vi "communication manager.vi"() -> ()   [LabVIEW 2018]
uses:
  communication-manager/socket REP/socket REP.lvclass
  C:/Users/Denis/Desktop/S4CCS/S4CCS/communication-manager/Socket/Socket.lvclass
  communication-manager/socket SUB/socket SUB.lvclass
  communication-manager/socket PUB/socket PUB.lvclass
  communication-manager/RxTx/RxTx.lvclass
  <vilib>/addons/zeromq/zmq_context.lvclass
  communication-manager/Socket/Socket.lvclass
panel:
  out "error out":errorcluster
  in  "socket PUB.lvclass":refnum<class "socket PUB.lvclass">
  in  "socket SUB.lvclass":refnum<class "socket SUB.lvclass">
  in  "socket REP.lvclass":refnum<class "socket REP.lvclass">
  # "Communication Manager of S4CCS"
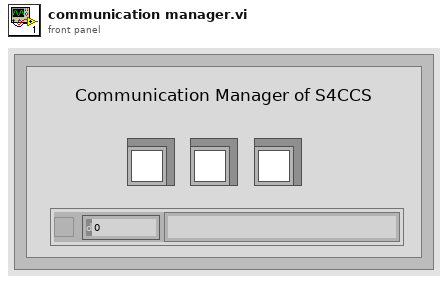
[diagram p1: front panel]
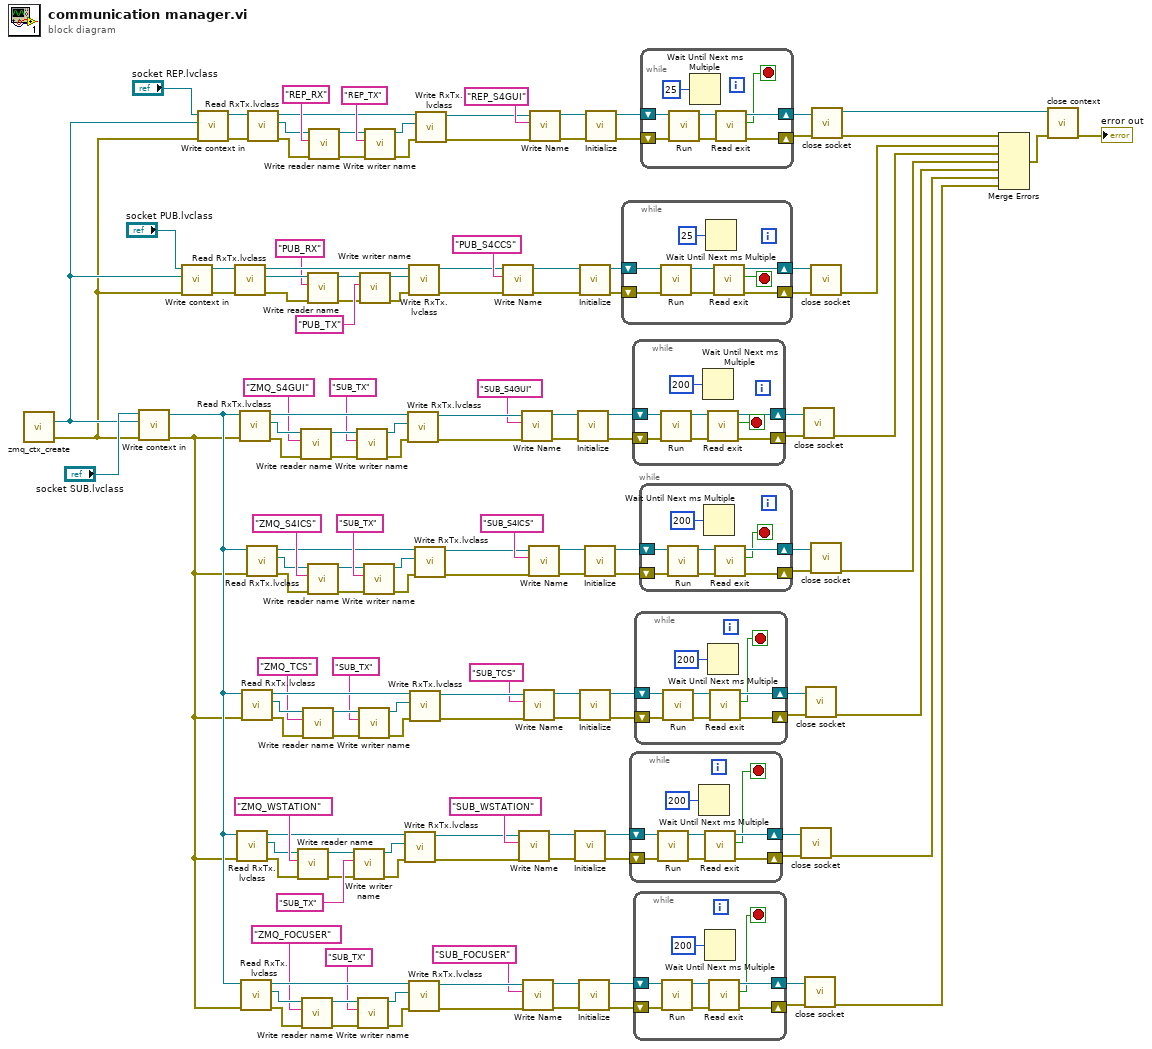
[diagram p0: block diagram]
diagram:
  n1 = call <vilib>:"zmq_ctx_create.vi"() -> ("error out"=w3:errorcluster, "context out"=w4:refnum<class "zmq_context.lvclass">)  [unwired: 4 in]
  n2 = call-dynamic "Write context in.vi"("error in (no error)"=w3, "zeromq.lvlib:ZeroMQ Context"=w4, "Socket in"="socket SUB.lvclass") -> ("error out"=w1:errorcluster, "Socket out"=w2:refnum<class "socket SUB.lvclass">)  [unwired: 7 in]
  n3 = call-dynamic "Write context in.vi"("error in (no error)"=w3, "zeromq.lvlib:ZeroMQ Context"=w4, "Socket in"="socket PUB.lvclass") -> ("error out"=w7:errorcluster, "Socket out"=w8:refnum<class "socket PUB.lvclass">)  [unwired: 7 in]
  n4 = call-dynamic "Write context in.vi"("error in (no error)"=w3, "zeromq.lvlib:ZeroMQ Context"=w4, "Socket in"="socket REP.lvclass") -> ("error out"=w10:errorcluster, "Socket out"=w11:refnum<class "socket REP.lvclass">)  [unwired: 7 in]
  n5 = call-dynamic "Read RxTx.lvclass.vi"("error in (no error)"=w7, "Socket in"=w8) -> ("error out"=w116:errorcluster, "RxTx.lvclass"=w120:refnum<class "RxTx.lvclass">, "Socket out"=w117:refnum<class "socket PUB.lvclass">)  [unwired: 7 in]
  n6 = call-dynamic "Read RxTx.lvclass.vi"("error in (no error)"=w1, "Socket in"=w2) -> ("error out"=w51:errorcluster, "RxTx.lvclass"=w55:refnum<class "RxTx.lvclass">, "Socket out"=w52:refnum<class "socket SUB.lvclass">)  [unwired: 7 in]
  n7 = call-dynamic "Read RxTx.lvclass.vi"("error in (no error)"=w1, "Socket in"=w2) -> ("error out"=w98:errorcluster, "RxTx.lvclass"=w94:refnum<class "RxTx.lvclass">, "Socket out"=w97:refnum<class "socket SUB.lvclass">)  [unwired: 7 in]
  n8 = call-dynamic "Read RxTx.lvclass.vi"("error in (no error)"=w1, "Socket in"=w2) -> ("error out"=w32:errorcluster, "RxTx.lvclass"=w28:refnum<class "RxTx.lvclass">, "Socket out"=w31:refnum<class "socket SUB.lvclass">)  [unwired: 7 in]
  n9 = call-dynamic "Read RxTx.lvclass.vi"("error in (no error)"=w1, "Socket in"=w2) -> ("error out"=w64:errorcluster, "RxTx.lvclass"=w60:refnum<class "RxTx.lvclass">, "Socket out"=w63:refnum<class "socket SUB.lvclass">)  [unwired: 7 in]
  n10 = call-dynamic "Read RxTx.lvclass.vi"("error in (no error)"=w1, "Socket in"=w2) -> ("error out"=w83:errorcluster, "RxTx.lvclass"=w87:refnum<class "RxTx.lvclass">, "Socket out"=w84:refnum<class "socket SUB.lvclass">)  [unwired: 7 in]
  n11 = call-dynamic "Read RxTx.lvclass.vi"("error in (no error)"=w10, "Socket in"=w11) -> ("error out"=w140:errorcluster, "RxTx.lvclass"=w144:refnum<class "RxTx.lvclass">, "Socket out"=w141:refnum<class "socket REP.lvclass">)  [unwired: 7 in]
  n12 = call-dynamic "Write reader name.vi"("error in (no error)"=w51, "RX name"="ZMQ_WSTATION" ("reader name"), "RxTx in"=w55) -> ("error out"=w50:errorcluster, "RxTx out"=w54:refnum<class "RxTx.lvclass">)  [unwired: 7 in]
  n13 = call-dynamic "Write reader name.vi"("error in (no error)"=w98, "RX name"="ZMQ_S4GUI" ("reader name"), "RxTx in"=w94) -> ("error out"=w99:errorcluster, "RxTx out"=w95:refnum<class "RxTx.lvclass">)  [unwired: 7 in]
  n14 = call-dynamic "Write reader name.vi"("error in (no error)"=w32, "RX name"="ZMQ_FOCUSER" ("reader name"), "RxTx in"=w28) -> ("error out"=w33:errorcluster, "RxTx out"=w29:refnum<class "RxTx.lvclass">)  [unwired: 7 in]
  n15 = call-dynamic "Write reader name.vi"("error in (no error)"=w64, "RX name"="ZMQ_TCS" ("reader name"), "RxTx in"=w60) -> ("error out"=w65:errorcluster, "RxTx out"=w61:refnum<class "RxTx.lvclass">)  [unwired: 7 in]
  n16 = call-dynamic "Write reader name.vi"("error in (no error)"=w116, "RX name"="PUB_RX" ("reader name"), "RxTx in"=w120) -> ("error out"=w115:errorcluster, "RxTx out"=w119:refnum<class "RxTx.lvclass">)  [unwired: 7 in]
  n17 = call-dynamic "Write reader name.vi"("error in (no error)"=w83, "RX name"="ZMQ_S4ICS" ("reader name"), "RxTx in"=w87) -> ("error out"=w82:errorcluster, "RxTx out"=w86:refnum<class "RxTx.lvclass">)  [unwired: 7 in]
  n18 = call-dynamic "Write reader name.vi"("error in (no error)"=w140, "RX name"="REP_RX" ("reader name"), "RxTx in"=w144) -> ("error out"=w139:errorcluster, "RxTx out"=w143:refnum<class "RxTx.lvclass">)  [unwired: 7 in]
  n19 = call-dynamic "Write writer name.vi"("error in (no error)"=w50, "Tx name"="SUB_TX" ("writer name"), "RxTx in"=w54) -> ("error out"=w49:errorcluster, "RxTx out"=w53:refnum<class "RxTx.lvclass">)  [unwired: 7 in]
  n20 = call-dynamic "Write writer name.vi"("error in (no error)"=w99, "Tx name"="SUB_TX" ("writer name"), "RxTx in"=w95) -> ("error out"=w100:errorcluster, "RxTx out"=w96:refnum<class "RxTx.lvclass">)  [unwired: 7 in]
  n21 = call-dynamic "Write writer name.vi"("error in (no error)"=w33, "Tx name"="SUB_TX" ("writer name"), "RxTx in"=w29) -> ("error out"=w34:errorcluster, "RxTx out"=w30:refnum<class "RxTx.lvclass">)  [unwired: 7 in]
  n22 = call-dynamic "Write writer name.vi"("error in (no error)"=w65, "Tx name"="SUB_TX" ("writer name"), "RxTx in"=w61) -> ("error out"=w66:errorcluster, "RxTx out"=w62:refnum<class "RxTx.lvclass">)  [unwired: 7 in]
  n23 = call-dynamic "Write writer name.vi"("error in (no error)"=w115, "Tx name"="PUB_TX" ("writer name"), "RxTx in"=w119) -> ("error out"=w114:errorcluster, "RxTx out"=w118:refnum<class "RxTx.lvclass">)  [unwired: 7 in]
  n24 = call-dynamic "Write writer name.vi"("error in (no error)"=w82, "Tx name"="SUB_TX" ("writer name"), "RxTx in"=w86) -> ("error out"=w81:errorcluster, "RxTx out"=w85:refnum<class "RxTx.lvclass">)  [unwired: 7 in]
  n25 = call-dynamic "Write writer name.vi"("error in (no error)"=w139, "Tx name"="REP_TX" ("writer name"), "RxTx in"=w143) -> ("error out"=w138:errorcluster, "RxTx out"=w142:refnum<class "RxTx.lvclass">)  [unwired: 7 in]
  n26 = call-dynamic "Write RxTx.lvclass.vi"("error in (no error)"=w49, "RxTx.lvclass"=w53, "Socket in"=w52) -> ("error out"=w46:errorcluster, "Socket out"=w47:refnum<class "socket SUB.lvclass">)  [unwired: 7 in]
  n27 = call-dynamic "Write RxTx.lvclass.vi"("error in (no error)"=w100, "RxTx.lvclass"=w96, "Socket in"=w97) -> ("error out"=w103:errorcluster, "Socket out"=w102:refnum<class "socket SUB.lvclass">)  [unwired: 7 in]
  n28 = call-dynamic "Write RxTx.lvclass.vi"("error in (no error)"=w114, "RxTx.lvclass"=w118, "Socket in"=w117) -> ("error out"=w12:errorcluster, "Socket out"=w13:refnum<class "socket PUB.lvclass">)  [unwired: 7 in]
  n29 = call-dynamic "Write RxTx.lvclass.vi"("error in (no error)"=w34, "RxTx.lvclass"=w30, "Socket in"=w31) -> ("error out"=w37:errorcluster, "Socket out"=w36:refnum<class "socket SUB.lvclass">)  [unwired: 7 in]
  n30 = call-dynamic "Write RxTx.lvclass.vi"("error in (no error)"=w66, "RxTx.lvclass"=w62, "Socket in"=w63) -> ("error out"=w69:errorcluster, "Socket out"=w68:refnum<class "socket SUB.lvclass">)  [unwired: 7 in]
  n31 = call-dynamic "Write RxTx.lvclass.vi"("error in (no error)"=w81, "RxTx.lvclass"=w85, "Socket in"=w84) -> ("error out"=w78:errorcluster, "Socket out"=w79:refnum<class "socket SUB.lvclass">)  [unwired: 7 in]
  n32 = call-dynamic "Write RxTx.lvclass.vi"("error in (no error)"=w138, "RxTx.lvclass"=w142, "Socket in"=w141) -> ("error out"=w135:errorcluster, "Socket out"=w136:refnum<class "socket REP.lvclass">)  [unwired: 7 in]
  n33 = call-dynamic "Write Name.vi"("error in (no error)"=w12, "Name"="PUB_S4CCS", "Socket in"=w13) -> ("error out"=w112:errorcluster, "Socket out"=w113:refnum<class "socket PUB.lvclass">)  [unwired: 7 in]
  n34 = call-dynamic "Write Name.vi"("error in (no error)"=w46, "Name"="SUB_WSTATION", "Socket in"=w47) -> ("error out"=w20:errorcluster, "Socket out"=w21:refnum<class "socket SUB.lvclass">)  [unwired: 7 in]
  n35 = call-dynamic "Write Name.vi"("error in (no error)"=w103, "Name"="SUB_S4GUI", "Socket in"=w102) -> ("error out"=w18:errorcluster, "Socket out"=w19:refnum<class "socket SUB.lvclass">)  [unwired: 7 in]
  n36 = call-dynamic "Write Name.vi"("error in (no error)"=w37, "Name"="SUB_FOCUSER", "Socket in"=w36) -> ("error out"=w14:errorcluster, "Socket out"=w15:refnum<class "socket SUB.lvclass">)  [unwired: 7 in]
  n37 = call-dynamic "Write Name.vi"("error in (no error)"=w69, "Name"="SUB_TCS", "Socket in"=w68) -> ("error out"=w24:errorcluster, "Socket out"=w25:refnum<class "socket SUB.lvclass">)  [unwired: 7 in]
  n38 = call-dynamic "Write Name.vi"("error in (no error)"=w78, "Name"="SUB_S4ICS", "Socket in"=w79) -> ("error out"=w22:errorcluster, "Socket out"=w23:refnum<class "socket SUB.lvclass">)  [unwired: 7 in]
  n39 = call-dynamic "Write Name.vi"("error in (no error)"=w135, "Name"="REP_S4GUI", "Socket in"=w136) -> ("error out"=w16:errorcluster, "Socket out"=w17:refnum<class "socket REP.lvclass">)  [unwired: 7 in]
  n40 = call-dynamic "Initialize.vi"("error in (no error)"=w20, "socket SUB in"=w21) -> ("error out"=w43:errorcluster, "socket SUB out"=w45:refnum<class "socket SUB.lvclass">)  [unwired: 8 in]
  n41 = call-dynamic "Initialize.vi"("error in (no error)"=w18, "socket SUB in"=w19) -> ("error out"=w106:errorcluster, "socket SUB out"=w104:refnum<class "socket SUB.lvclass">)  [unwired: 8 in]
  n42 = call-dynamic "Initialize.vi"("error in (no error)"=w14, "socket SUB in"=w15) -> ("error out"=w40:errorcluster, "socket SUB out"=w38:refnum<class "socket SUB.lvclass">)  [unwired: 8 in]
  n43 = call-dynamic "Initialize.vi"("error in (no error)"=w112, "socket PUB in"=w113) -> ("error out"=w109:errorcluster, "socket PUB out"=w111:refnum<class "socket PUB.lvclass">)  [unwired: 8 in]
  n44 = call-dynamic "Initialize.vi"("error in (no error)"=w24, "socket SUB in"=w25) -> ("error out"=w72:errorcluster, "socket SUB out"=w70:refnum<class "socket SUB.lvclass">)  [unwired: 8 in]
  n45 = call-dynamic "Initialize.vi"("error in (no error)"=w22, "socket SUB in"=w23) -> ("error out"=w75:errorcluster, "socket SUB out"=w77:refnum<class "socket SUB.lvclass">)  [unwired: 8 in]
  n46 = call-dynamic "Initialize.vi"("error in (no error)"=w16, "socket REP in"=w17) -> ("error out"=w132:errorcluster, "socket REP out"=w134:refnum<class "socket REP.lvclass">)  [unwired: 8 in]
  n47 = while {
    shift-right: [w151] -> w110
    shift-left: w111 -> [w155]
    shift-right: [w150] -> w108
    shift-left: w109 -> [w154]
    stop <- w149 stop-if-true
    n48 = call-dynamic "Run.vi"("error in (no error)"=w154, "socket PUB in"=w155) -> ("error out"=w153:errorcluster, "socket PUB out"=w152:refnum<class "socket PUB.lvclass">)  [unwired: 8 in]
    n49 = Wait Until Next ms Multiple(millisecond multiple=u32 25) -> ()  [unwired: 1 out]
    n50 = call-dynamic "Read exit.vi"("error in (no error)"=w153, "Socket in"=w152) -> ("error out"=w150:errorcluster, "exit"=w149:bool, "Socket out"=w151:refnum<class "socket PUB.lvclass">)  [unwired: 7 in]
  }
  n51 = while {
    shift-right: [w161] -> w44
    shift-left: w45 -> [w163]
    shift-right: [w158] -> w42
    shift-left: w43 -> [w160]
    stop <- w157 stop-if-true
    n52 = call-dynamic "Run.vi"("error in (no error)"=w160, "socket SUB in"=w163) -> ("error out"=w159:errorcluster, "socket SUB out"=w162:refnum<class "socket SUB.lvclass">)  [unwired: 8 in]
    n53 = Wait Until Next ms Multiple(millisecond multiple=u32 200) -> ()  [unwired: 1 out]
    n54 = call-dynamic "Read exit.vi"("error in (no error)"=w159, "Socket in"=w162) -> ("error out"=w158:errorcluster, "exit"=w157:bool, "Socket out"=w161:refnum<class "socket SUB.lvclass">)  [unwired: 7 in]
  }
  n55 = while {
    shift-right: [w169] -> w105
    shift-left: w104 -> [w171]
    shift-right: [w166] -> w107
    shift-left: w106 -> [w168]
    stop <- w165 stop-if-true
    n56 = call-dynamic "Run.vi"("error in (no error)"=w168, "socket SUB in"=w171) -> ("error out"=w167:errorcluster, "socket SUB out"=w170:refnum<class "socket SUB.lvclass">)  [unwired: 8 in]
    n57 = Wait Until Next ms Multiple(millisecond multiple=u32 200) -> ()  [unwired: 1 out]
    n58 = call-dynamic "Read exit.vi"("error in (no error)"=w167, "Socket in"=w170) -> ("error out"=w166:errorcluster, "exit"=w165:bool, "Socket out"=w169:refnum<class "socket SUB.lvclass">)  [unwired: 7 in]
  }
  n59 = while {
    shift-right: [w177] -> w39
    shift-left: w38 -> [w179]
    shift-right: [w174] -> w41
    shift-left: w40 -> [w176]
    stop <- w173 stop-if-true
    n60 = call-dynamic "Run.vi"("error in (no error)"=w176, "socket SUB in"=w179) -> ("error out"=w175:errorcluster, "socket SUB out"=w178:refnum<class "socket SUB.lvclass">)  [unwired: 8 in]
    n61 = Wait Until Next ms Multiple(millisecond multiple=u32 200) -> ()  [unwired: 1 out]
    n62 = call-dynamic "Read exit.vi"("error in (no error)"=w175, "Socket in"=w178) -> ("error out"=w174:errorcluster, "exit"=w173:bool, "Socket out"=w177:refnum<class "socket SUB.lvclass">)  [unwired: 7 in]
  }
  n63 = while {
    shift-right: [w185] -> w71
    shift-left: w70 -> [w187]
    shift-right: [w182] -> w73
    shift-left: w72 -> [w184]
    stop <- w181 stop-if-true
    n64 = call-dynamic "Run.vi"("error in (no error)"=w184, "socket SUB in"=w187) -> ("error out"=w183:errorcluster, "socket SUB out"=w186:refnum<class "socket SUB.lvclass">)  [unwired: 8 in]
    n65 = Wait Until Next ms Multiple(millisecond multiple=u32 200) -> ()  [unwired: 1 out]
    n66 = call-dynamic "Read exit.vi"("error in (no error)"=w183, "Socket in"=w186) -> ("error out"=w182:errorcluster, "exit"=w181:bool, "Socket out"=w185:refnum<class "socket SUB.lvclass">)  [unwired: 7 in]
  }
  n67 = while {
    shift-right: [w193] -> w76
    shift-left: w77 -> [w195]
    shift-right: [w190] -> w74
    shift-left: w75 -> [w192]
    stop <- w189 stop-if-true
    n68 = call-dynamic "Run.vi"("error in (no error)"=w192, "socket SUB in"=w195) -> ("error out"=w191:errorcluster, "socket SUB out"=w194:refnum<class "socket SUB.lvclass">)  [unwired: 8 in]
    n69 = Wait Until Next ms Multiple(millisecond multiple=u32 200) -> ()  [unwired: 1 out]
    n70 = call-dynamic "Read exit.vi"("error in (no error)"=w191, "Socket in"=w194) -> ("error out"=w190:errorcluster, "exit"=w189:bool, "Socket out"=w193:refnum<class "socket SUB.lvclass">)  [unwired: 7 in]
  }
  n71 = while {
    shift-right: [w201] -> w133
    shift-left: w134 -> [w203]
    shift-right: [w198] -> w131
    shift-left: w132 -> [w200]
    stop <- w197 stop-if-true
    n72 = call-dynamic "Run.vi"("error in (no error)"=w200, "socket REP in"=w203) -> ("error out"=w199:errorcluster, "socket REP out"=w202:refnum<class "socket REP.lvclass">)  [unwired: 8 in]
    n73 = Wait Until Next ms Multiple(millisecond multiple=u32 25) -> ()  [unwired: 1 out]
    n74 = call-dynamic "Read exit.vi"("error in (no error)"=w199, "Socket in"=w202) -> ("error out"=w198:errorcluster, "exit"=w197:bool, "Socket out"=w201:refnum<class "socket REP.lvclass">)  [unwired: 7 in]
  }
  n75 = call "close socket.vi"("error in (no error)"=w42, "Socket in"=w44) -> ("error out"=w122:errorcluster)  [unwired: 8 in, 1 out]
  n76 = call "close socket.vi"("error in (no error)"=w107, "Socket in"=w105) -> ("error out"=w128:errorcluster)  [unwired: 8 in, 1 out]
  n77 = call "close socket.vi"("error in (no error)"=w41, "Socket in"=w39) -> ("error out"=w121:errorcluster)  [unwired: 8 in, 1 out]
  n78 = call "close socket.vi"("error in (no error)"=w73, "Socket in"=w71) -> ("error out"=w123:errorcluster)  [unwired: 8 in, 1 out]
  n79 = call "close socket.vi"("error in (no error)"=w108, "Socket in"=w110) -> ("error out"=w129:errorcluster)  [unwired: 8 in, 1 out]
  n80 = call "close socket.vi"("error in (no error)"=w74, "Socket in"=w76) -> ("error out"=w124:errorcluster)  [unwired: 8 in, 1 out]
  n81 = call "close socket.vi"("error in (no error)"=w131, "Socket in"=w133) -> ("error out"=w130:errorcluster, "Socket out"=w126:refnum<class "socket REP.lvclass">)  [unwired: 8 in]
  n82 = Merge Errors(w130, w129, w128, w124, w123, w122, w121) -> (w127:errorcluster)
  n83 = call-dynamic "close context.vi"("error in (no error)"=w127, "Socket in"=w126) -> ("error out"=→"error out":errorcluster)  [unwired: 8 in, 1 out]
